vi "Concatenate Paths.vi"(1 "Autos":T10(array[cluster]) {"Fields"."Overrides"."Angle Override" step=5.0; "Fields"."Overrides"."Velocity Override" step=5.0; "Fields"."Overrides"."Angular Override" step=5.0; "Fields"."Angular Limits"."Jerk (deg/s^3)" min=0.0 step=1.0; "Fields"."Angular Limits"."Accel (deg/s^2)" min=0.0; "Fields"."Angular Limits"."Velocity (deg/s)" min=0.0}) -> (0 "Auto":T1)   [LabVIEW 2020]
uses:
  submodules/bordeaux-pathinator/Bordeaux/Types/Single Cmd Info.ctl
  <vilib>/picture/picture.llb/imagedata.ctl
  submodules/bordeaux-pathinator/Bordeaux/Types/Trajectory Data.ctl
  submodules/bordeaux-pathinator/Bordeaux/Types/Segment Type.ctl
  submodules/bordeaux-pathinator/Bordeaux/Types/Overrides.ctl
  submodules/bordeaux-pathinator/Bordeaux/Types/Angluar Limits.ctl
  submodules/bordeaux-pathinator/Bordeaux/Types/Drive Type.ctl
  submodules/bordeaux-pathinator/Bordeaux/Types/Path Type.ctl
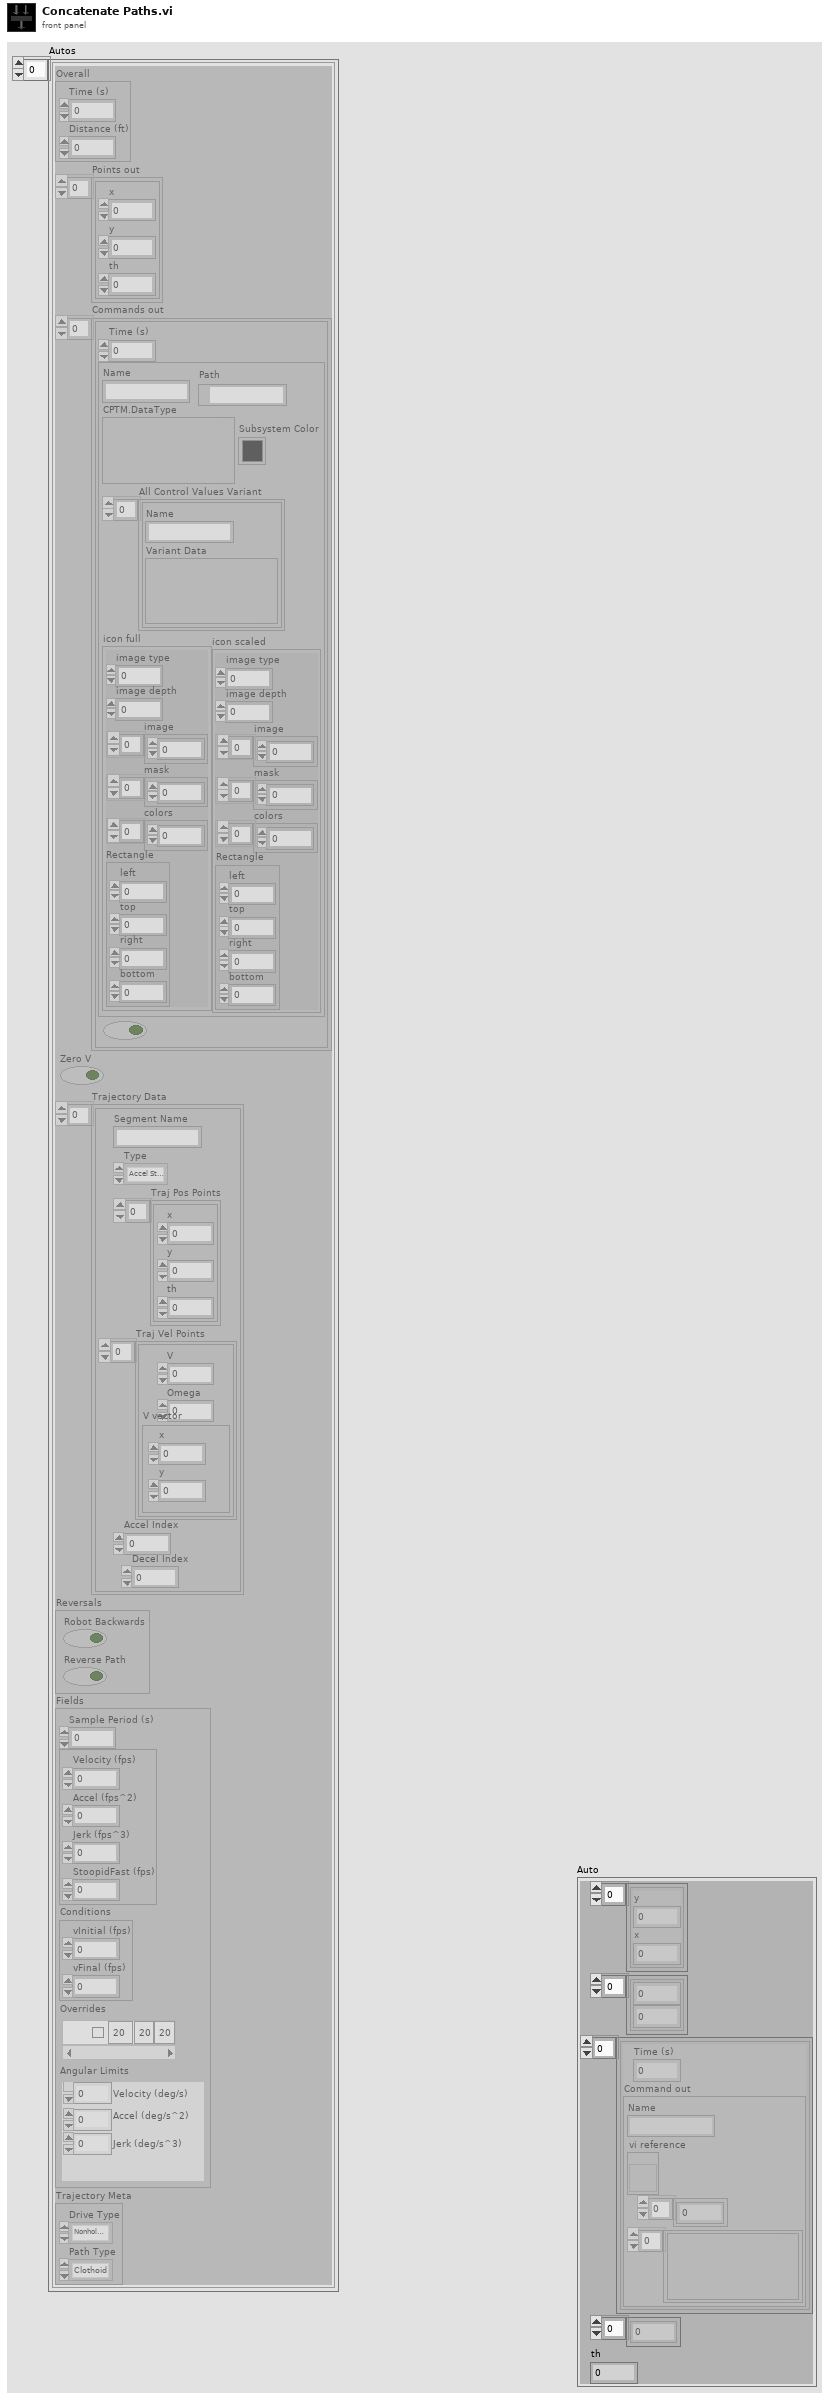
[diagram p1: front panel]
types:
  T1 = cluster{cluster{"y":dbl, "x":dbl}[], cluster{dbl, dbl}[], cluster{"Time (s)":dbl, "Command out":cluster{"Name":string, "vi reference":refnum<vi>, i32[], variant[]}}[], i32[], "th":dbl}
  T2 = typedef "Single Cmd Info.ctl" = cluster{"Name":string, "CPTM.DataType":variant, "All Control Values Variant":cluster{"Name":string, "Variant Data":variant}[], "icon full":T3, "icon scaled":T3, "Path":path, "Subsystem Color":u32}
  T3 = typedef "imagedata.ctl" = cluster{"image type":i32, "image depth":i32, "image":u8[], "mask":u8[], "colors":u32[], "Rectangle":cluster{"left":i16, "top":i16, "right":i16, "bottom":i16}}
  T4 = typedef "Trajectory Data.ctl" = cluster{"Segment Name":string, "Type":T5, "Traj Pos Points":cluster{"x":dbl, "y":dbl, "th":dbl}[], "Traj Vel Points":cluster{"V":dbl, "Omega":dbl, "V vector":cluster{"y":dbl, "x":dbl}}[], "Accel Index":i32, "Decel Index":i32}[]
  T5 = typedef "Segment Type.ctl" = enum16{"Accel Straight", "Const Straight", "Blend", "Circle", "Bezier"}
  T6 = typedef "Overrides.ctl" = cluster{"Count":string, "Angular Override":dbl, "Enabled?":bool, "Velocity Override":dbl, "Angle Override":dbl}[]
  T7 = typedef "Angluar Limits.ctl" = cluster{"Velocity (deg/s)":dbl, "Accel (deg/s^2)":dbl, "Jerk (deg/s^3)":dbl}
  T8 = typedef "Drive Type.ctl" = enum16{"Nonholonomic", "Holonomic"}
  T9 = typedef "Path Type.ctl" = enum16{"Clothoid", "Bezier"}
  T10 = cluster{"Overall":cluster{"Time (s)":dbl, "Distance (ft)":dbl}, "Points out":cluster{"x":dbl, "y":dbl, "th":dbl}[], "Commands out":cluster{"Time (s)":dbl, T2, bool}[], "Zero V":bool, "Trajectory Data":T4, "Reversals":cluster{"Robot Backwards":bool, "Reverse Path":bool}, "Fields":cluster{"Sample Period (s)":dbl, cluster{"Velocity (fps)":dbl, "Accel (fps^2)":dbl, "Jerk (fps^3)":dbl, "StoopidFast (fps)":dbl}, "Conditions":cluster{"vInitial (fps)":dbl, "vFinal (fps)":dbl}, "Overrides":T6, "Angular Limits":T7}, "Trajectory Meta":cluster{"Drive Type":T8, "Path Type":T9}}[]
  T11 = cluster{"Robot Backwards":bool, "Reverse Path":bool}
  T12 = cluster{"V":dbl, "Omega":dbl, "V vector":cluster{"y":dbl, "x":dbl}}[]
  T13 = cluster{"Segment Name":string, "Type":T5, "Traj Pos Points":cluster{"x":dbl, "y":dbl, "th":dbl}[], "Traj Vel Points":cluster{"V":dbl, "Omega":dbl, "V vector":cluster{"y":dbl, "x":dbl}}[], "Accel Index":i32, "Decel Index":i32}
  T14 = cluster{"Name":string, "vi reference":refnum<vi>, i32[], variant[]}
  T15 = cluster{"Time (s)":dbl, "Command out":cluster{"Name":string, "vi reference":refnum<vi>, i32[], variant[]}}
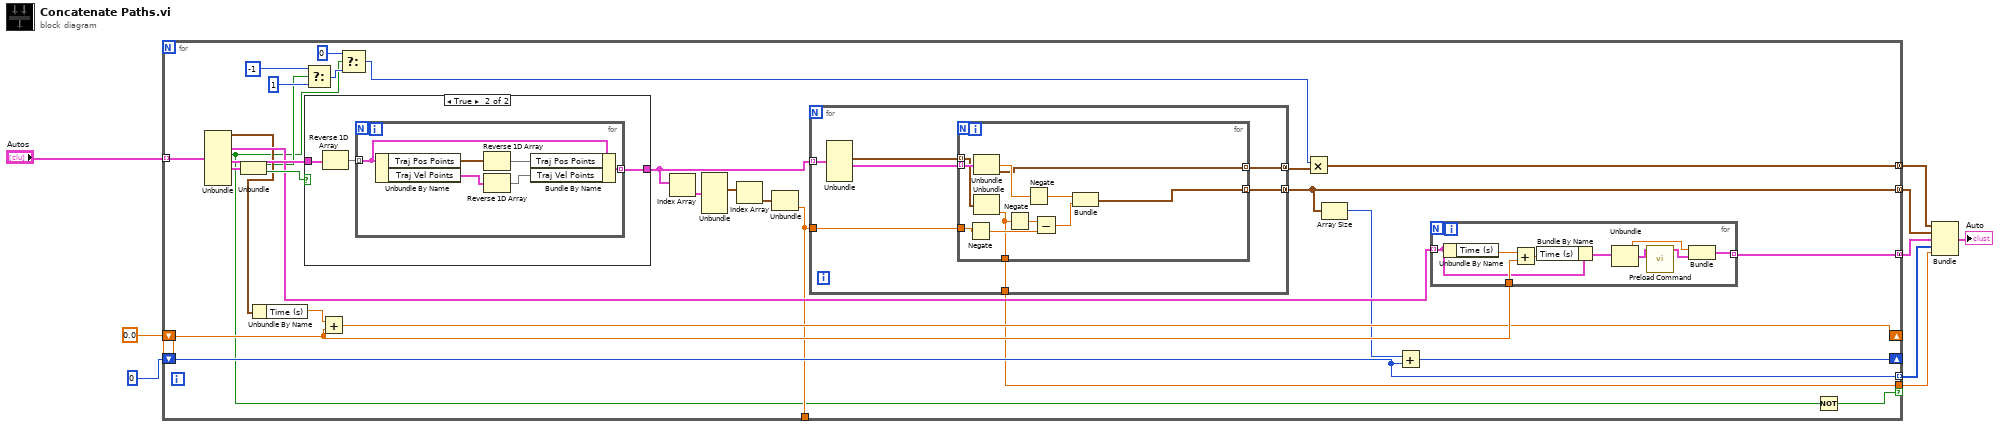
[diagram p0: block diagram]
diagram:
  n1 = for {
    tunnel: "Autos" -> [w39] mode=indexing
    shift-right: [w20] -> _
    shift-left: 0.0 -> [w21]
    tunnel: [w25] -> w6 mode=concatenating
    tunnel: [w18] -> w5 mode=concatenating
    tunnel: [w19] -> w4 mode=concatenating
    shift-right: [w16] -> _
    shift-left: 0 -> [w15]
    tunnel: [w15] -> w3 mode=indexing
    tunnel: [w14] -> w2 if=w10
    tunnel: [w12] -> _
    n2 = Unbundle(w39) -> ("Overall"=w23:cluster{"Time (s)":dbl, "Distance (ft)":dbl}, "Commands out"=w24:cluster{"Time (s)":dbl, T2, bool}[], "Zero V"=w11:bool, "Trajectory Data"=w37:T4, "Reversals"=w38:T11)  [unwired: 3 out]
    n3 = Unbundle(w38) -> ("Robot Backwards"=w13:bool, "Reverse Path"=w36:bool)
    n4 = Unbundle By Name(w23) -> ("Time (s)"=w22:dbl)
    n5 = case shown="True" w36 {
      tunnel: w37 -> [w67 w70]
      tunnel: [w67 w68] -> w32
      frame False {
      }
      frame True {
        n6 = Reverse 1D Array(array=w70) -> (reversed array=w69:T4)
        n7 = for {
          tunnel: w69 -> [w76] mode=indexing
          tunnel: [w71] -> w68 mode=indexing
          n8 = Unbundle By Name(w76) -> ("Traj Pos Points"=w75:cluster{"x":dbl, "y":dbl, "th":dbl}[], "Traj Vel Points"=w73:T12)
          n9 = Reverse 1D Array(array=w75) -> (reversed array=w74:cluster{"x":dbl, "y":dbl, "th":dbl}[])
          n10 = Reverse 1D Array(array=w73) -> (reversed array=w72:T12)
          n11 = Bundle By Name(cluster=w76, "Traj Pos Points"=w74, "Traj Vel Points"=w72) -> (w71:T13)
        }
      }
    }
    n12 = Select(t=-1, s=w13, f=1) -> (s? t:f=w28:i32)
    n13 = Add(x=w22, y=w21) -> (x+y=w20:dbl)
    n14 = Select(t=0, s=w11, f=w28) -> (s? t:f=w26:i32)
    n15 = Index Array(array=w32) -> (element=w31:T13)  [unwired: 1 in]
    n16 = Unbundle(w31) -> ("Traj Pos Points"=w30:cluster{"x":dbl, "y":dbl, "th":dbl}[])  [unwired: 5 out]
    n17 = Index Array(array=w30) -> (element=w29:cluster{"x":dbl, "y":dbl, "th":dbl})  [unwired: 1 in]
    n18 = Unbundle(w29) -> ("th"=w12:dbl)  [unwired: 2 out]
    n19 = for {
      tunnel: w32 -> [w55] mode=indexing
      tunnel: [w54] -> w33 mode=concatenating
      tunnel: [w53] -> w18 mode=concatenating
      tunnel: w12 -> [w50]
      tunnel: [w49] -> w14
      # "/shrug"
      n20 = Unbundle(w55) -> ("Traj Pos Points"=w51:cluster{"x":dbl, "y":dbl, "th":dbl}[], "Traj Vel Points"=w52:T12)  [unwired: 4 out]
      n21 = for {
        tunnel: w52 -> [w66] mode=indexing
        tunnel: [w58] -> w54 mode=indexing
        tunnel: [w65] -> w53 mode=indexing
        tunnel: w51 -> [w64] mode=indexing
        tunnel: w50 -> [w61]
        tunnel: [w56] -> w49
        n22 = Negate(x=w61) -> (-x=w59:dbl)
        n23 = Unbundle(w66) -> ("Omega"=w62:dbl, "V vector"=w58:cluster{"y":dbl, "x":dbl})  [unwired: 1 out]
        n24 = Unbundle(w64) -> ("th"=w56:dbl)  [unwired: 2 out]
        n25 = Negate(x=w56) -> (-x=w57:dbl)
        n26 = Negate(x=w62) -> (-x=w60:dbl)
        n27 = Subtract(x=w57, y=w59) -> (x-y=w63:dbl)
        n28 = Bundle(w60, w63) -> (w65:cluster{dbl, dbl})  [unwired: 1 in]
      }
    }
    n29 = Multiply(x=w26, y=w33) -> (x*y=w25:cluster{"y":dbl, "x":dbl}[])
    n30 = Array Size(array=w18) -> (size(s)=w17:i32)
    n31 = Add(x=w17, y=w15) -> (x+y=w16:i32)
    n32 = for {
      tunnel: w24 -> [w45] mode=indexing
      tunnel: w21 -> [w47]
      tunnel: [w43] -> w19 mode=indexing
      n33 = Unbundle By Name(w45) -> ("Time (s)"=w48:dbl)
      n34 = Add(x=w48, y=w47) -> (x+y=w46:dbl)
      n35 = Bundle By Name(cluster=w45, "Time (s)"=w46) -> (w44:cluster{"Time (s)":dbl, T2, bool})
      n36 = Unbundle(w44) -> ("Time (s)"=w41:dbl, w42:T2)  [unwired: 1 out]
      n37 = call "Preload Command.vi"("Command"=w42) -> ("Command out"=w40:T14)  [unwired: 10 in]
      n38 = Bundle("Time (s)"=w41, "Command out"=w40) -> (w43:T15)  [unwired: 1 in]
    }
    n39 = Not(x=w11) -> (.not. x?=w10:bool)
  }
  n40 = Bundle(w6, w5, w4, w3, "th"=w2) -> (→"Auto":T1)  [unwired: 1 in]
